vi "phase_josa.vi"(1 "beam cluster":T1 {"wavelength (in m)" format="%.2f"; "represented height (in m)" format="%.2f"; "represented width (in m)" format="%.2f"; "amplitude matrix" format="%.2f"}) -> (0 "phase matrix":dbl[][](array[numeric]) format="%.2f")   [LabVIEW 2015]
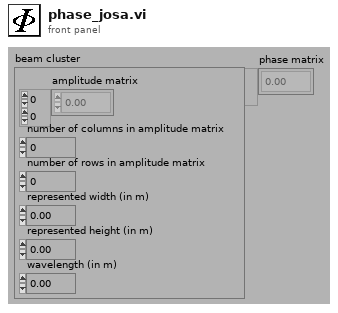
[diagram p1: front panel]
types:
  T1 = cluster{"amplitude matrix":cdb[][], "number of columns in amplitude matrix":i32, "number of rows in amplitude matrix":i32, "represented width (in m)":dbl, "represented height (in m)":dbl, "wavelength (in m)":dbl}
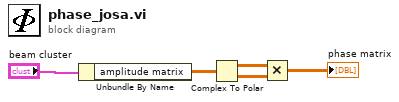
[diagram p0: block diagram]
diagram:
  n1 = Unbundle By Name("beam cluster") -> ("amplitude matrix"=w5:cdb[][])
  n2 = Complex To Polar(r * e^(i*theta)=w5) -> (r=w2:dbl[][], theta=w3:dbl[][])
  n3 = Multiply(x=w2, y=w3) -> (x*y=→"phase matrix":dbl[][])
